vi "Build Relative Process VI Path.vi"(3 "Rel Path":string) -> (1 "Full Path Out":path)   [LabVIEW 2014, in "Config Data.lvlib" / "Config Data.lvclass"]
uses:
  Config Data.lvclass
  Path Utilities/Path Utilities.lvlib
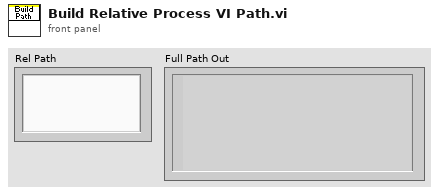
[diagram p1: front panel]
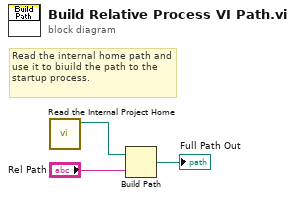
[diagram p0: block diagram]
diagram:
  # "Read the internal home path and use it to biuild the path to the startup process."
  n1 = call "Read the Internal Project Home.vi"() -> ("Internal Home Path"=w1:path)  [unwired: 6 in, 1 out]
  n2 = Build Path(base path=w1, name or relative path="Rel Path") -> (appended path=→"Full Path Out":path)
